vi "20260313_BIOEN468_FinalDraft_Final.vi"() -> ()   [LabVIEW 2025]
uses:
  <vilib>/Analysis/NI_AAL_SigProc.lvlib
  <vilib>/Waveform/WDTOps.llb/WDT Get Waveform Subset DBL.vi
  <vilib>/express/express analysis/Spectral/Block/exnSpectralBlock spectral measurements power poly.vi
  <vilib>/express/express analysis/Spectral/XNode/ExpressSpectralMeasurementsBlockNode.xnode
  <vilib>/Analysis/NI_AALBase.lvlib
  <vilib>/Analysis/baseanly.llb/Mean (DBL).vi
  <vilib>/express/express analysis/Spectral/Block/exnSpectralBlock spectral measurements power WFM.vi
  <vilib>/Waveform/WDTOps.llb/WDT Get XY Value DBL.vi
panel:
  out "Array 2":dbl[](array[numeric])
  out "Array":dbl[](array[numeric])
  out "Post truncation filtered top power spectrum":dbl[](graph)
  out "Post truncation filtered bottom power spectrum":dbl[](graph)
  out "Adventitious Lung Sound Detected":bool
  in  "threshold":dbl format="%.8f"
  out "# found":i32
  out "Bottom magnitudes":dbl[](graph)
  out "Top magnitudes":dbl[](graph)
  out "Subtracted magnitudes":dbl[](graph)
  out "Final Subtracted Power Spectrum":dbl[](graph)
  out "Truncated Waveform Top":waveform(dbl)(graph)
  in  "duration(s)  bottom":dbl
  out "sample rate (S/s) 2":dbl
  in  "File bottom":path
  in  "File top":path
  out "sample rate (S/s) 3":dbl
  in  "stop":bool
  in  "duration(s) top":dbl
  out "Truncated Waveform Bottom":waveform(dbl)(graph)
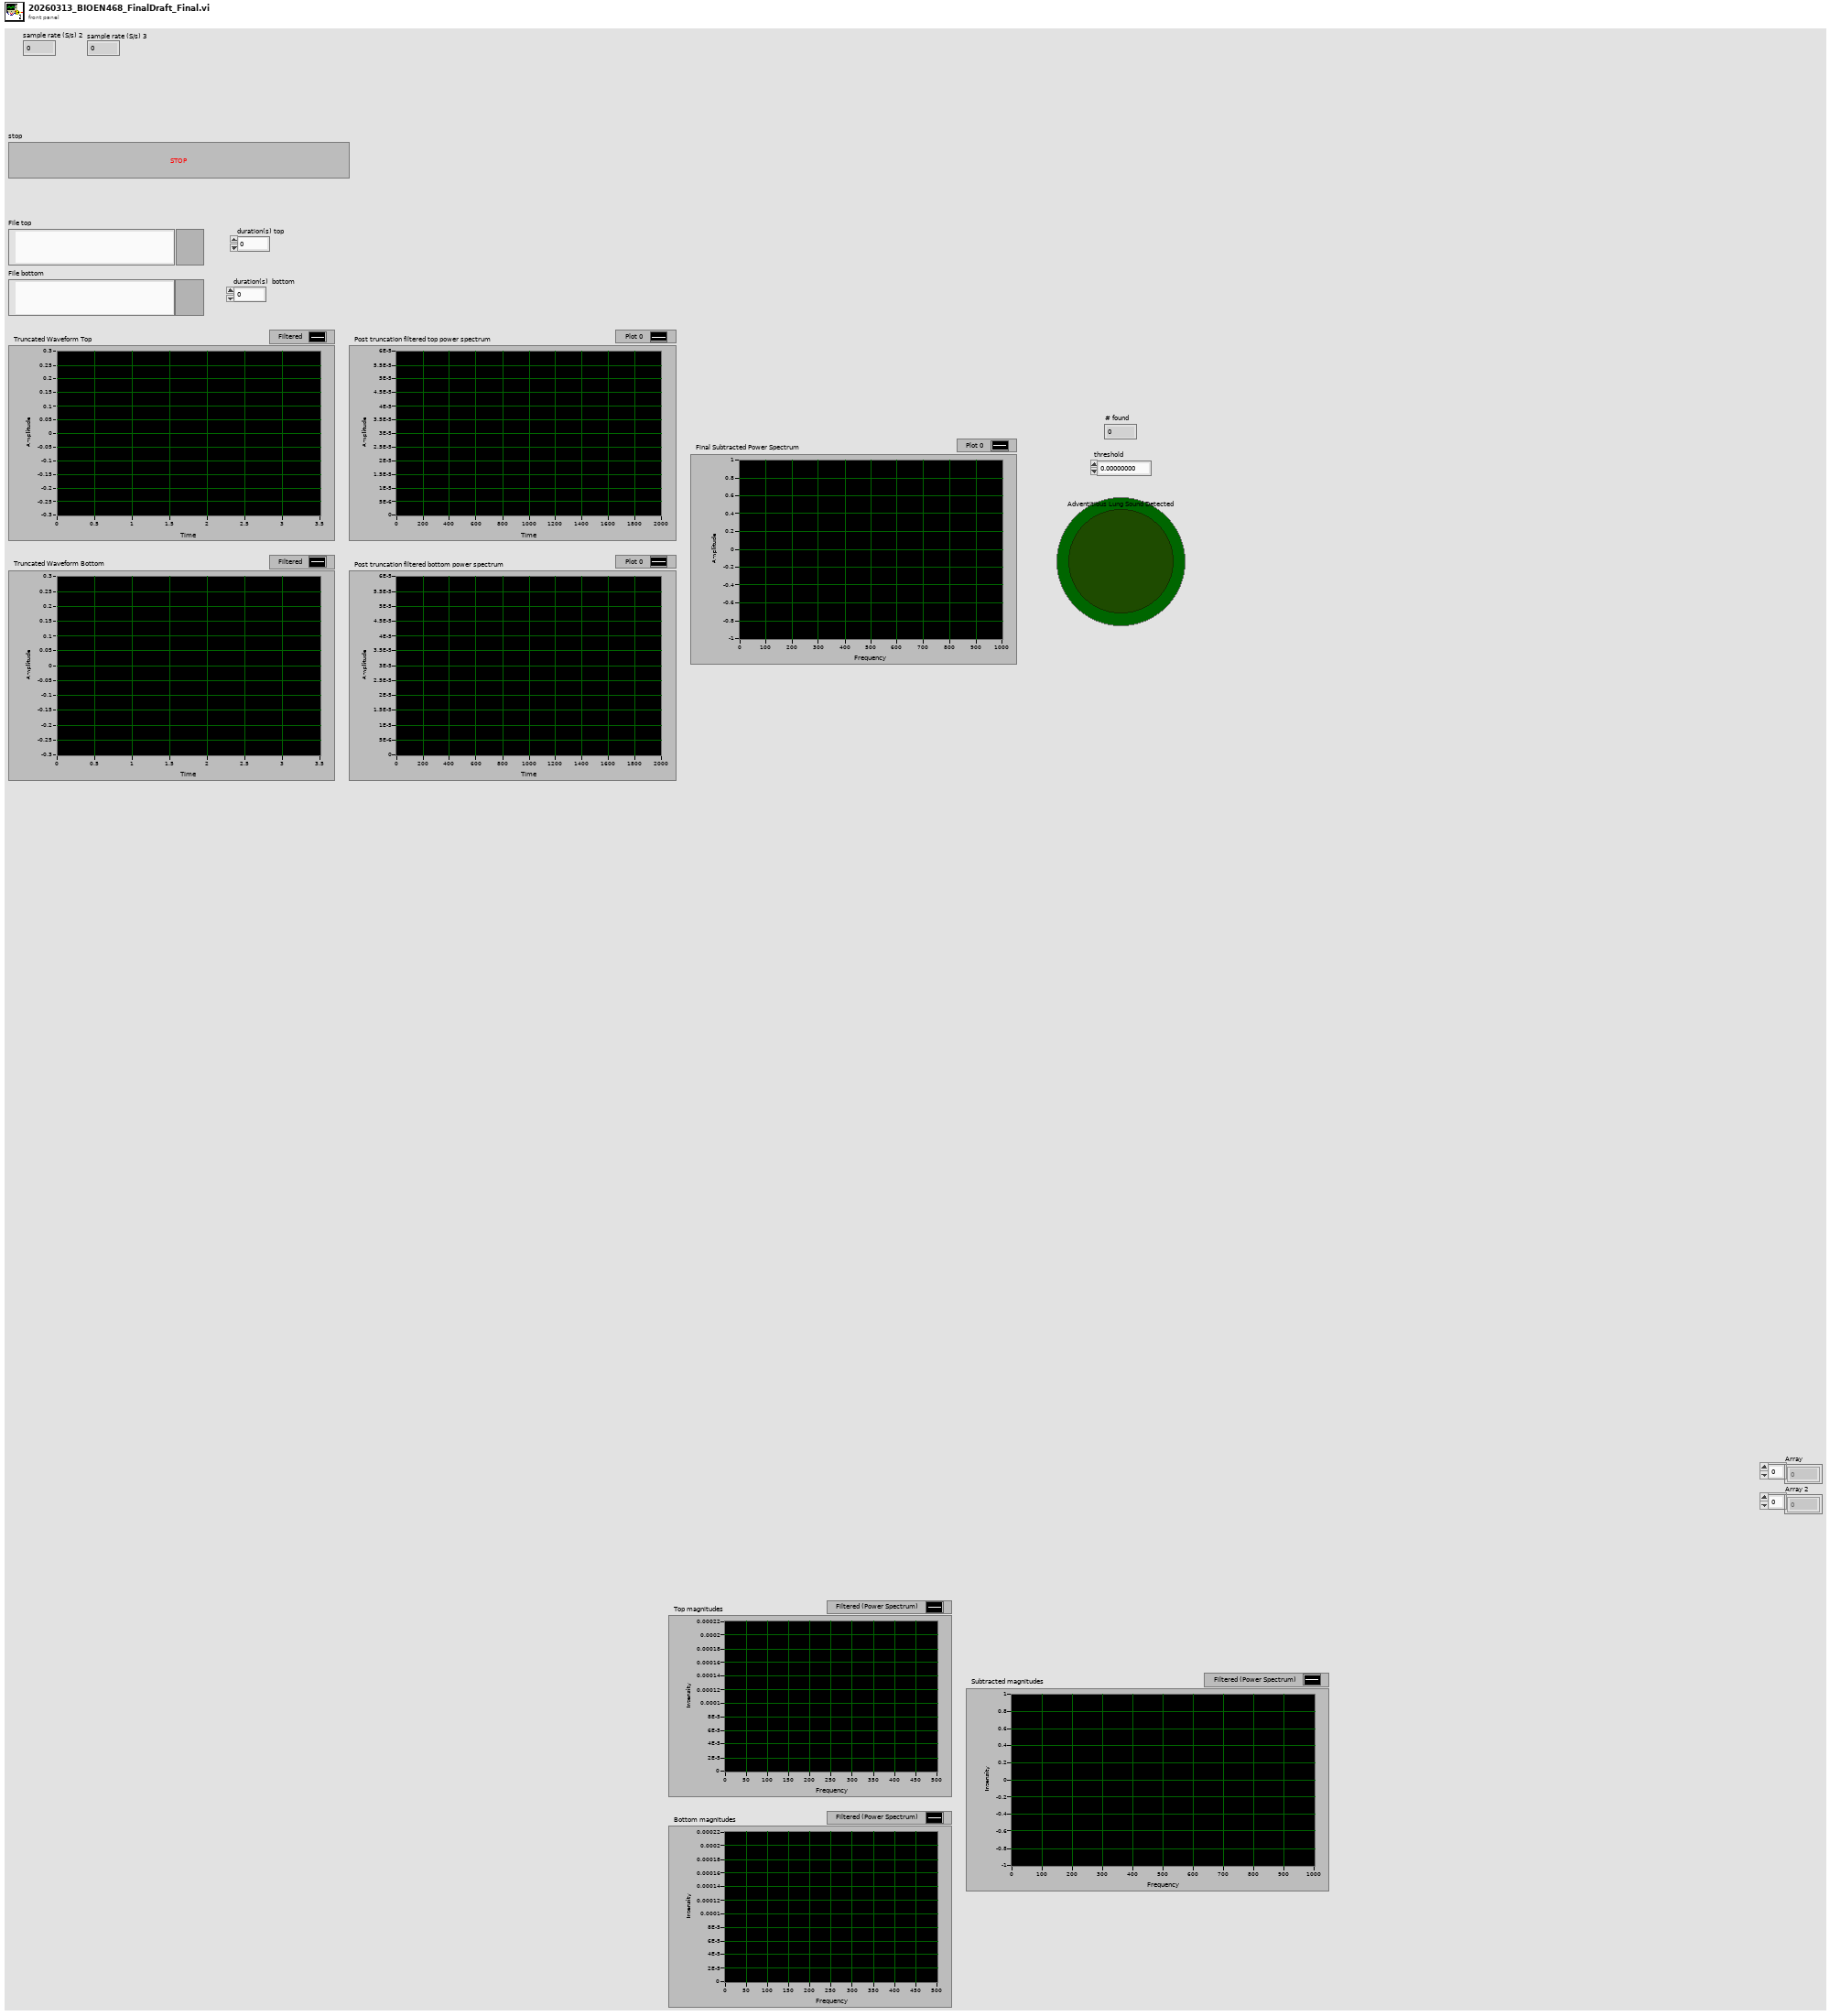
[diagram p1: front panel]
types:
  T1 = cluster{"averaging mode":u16, "weighting mode":u16, "number of averages":u32}
  T2 = cluster{"dB On (F)":bool, "unwrap phase (F)":bool, "convert to degree (F)":bool}
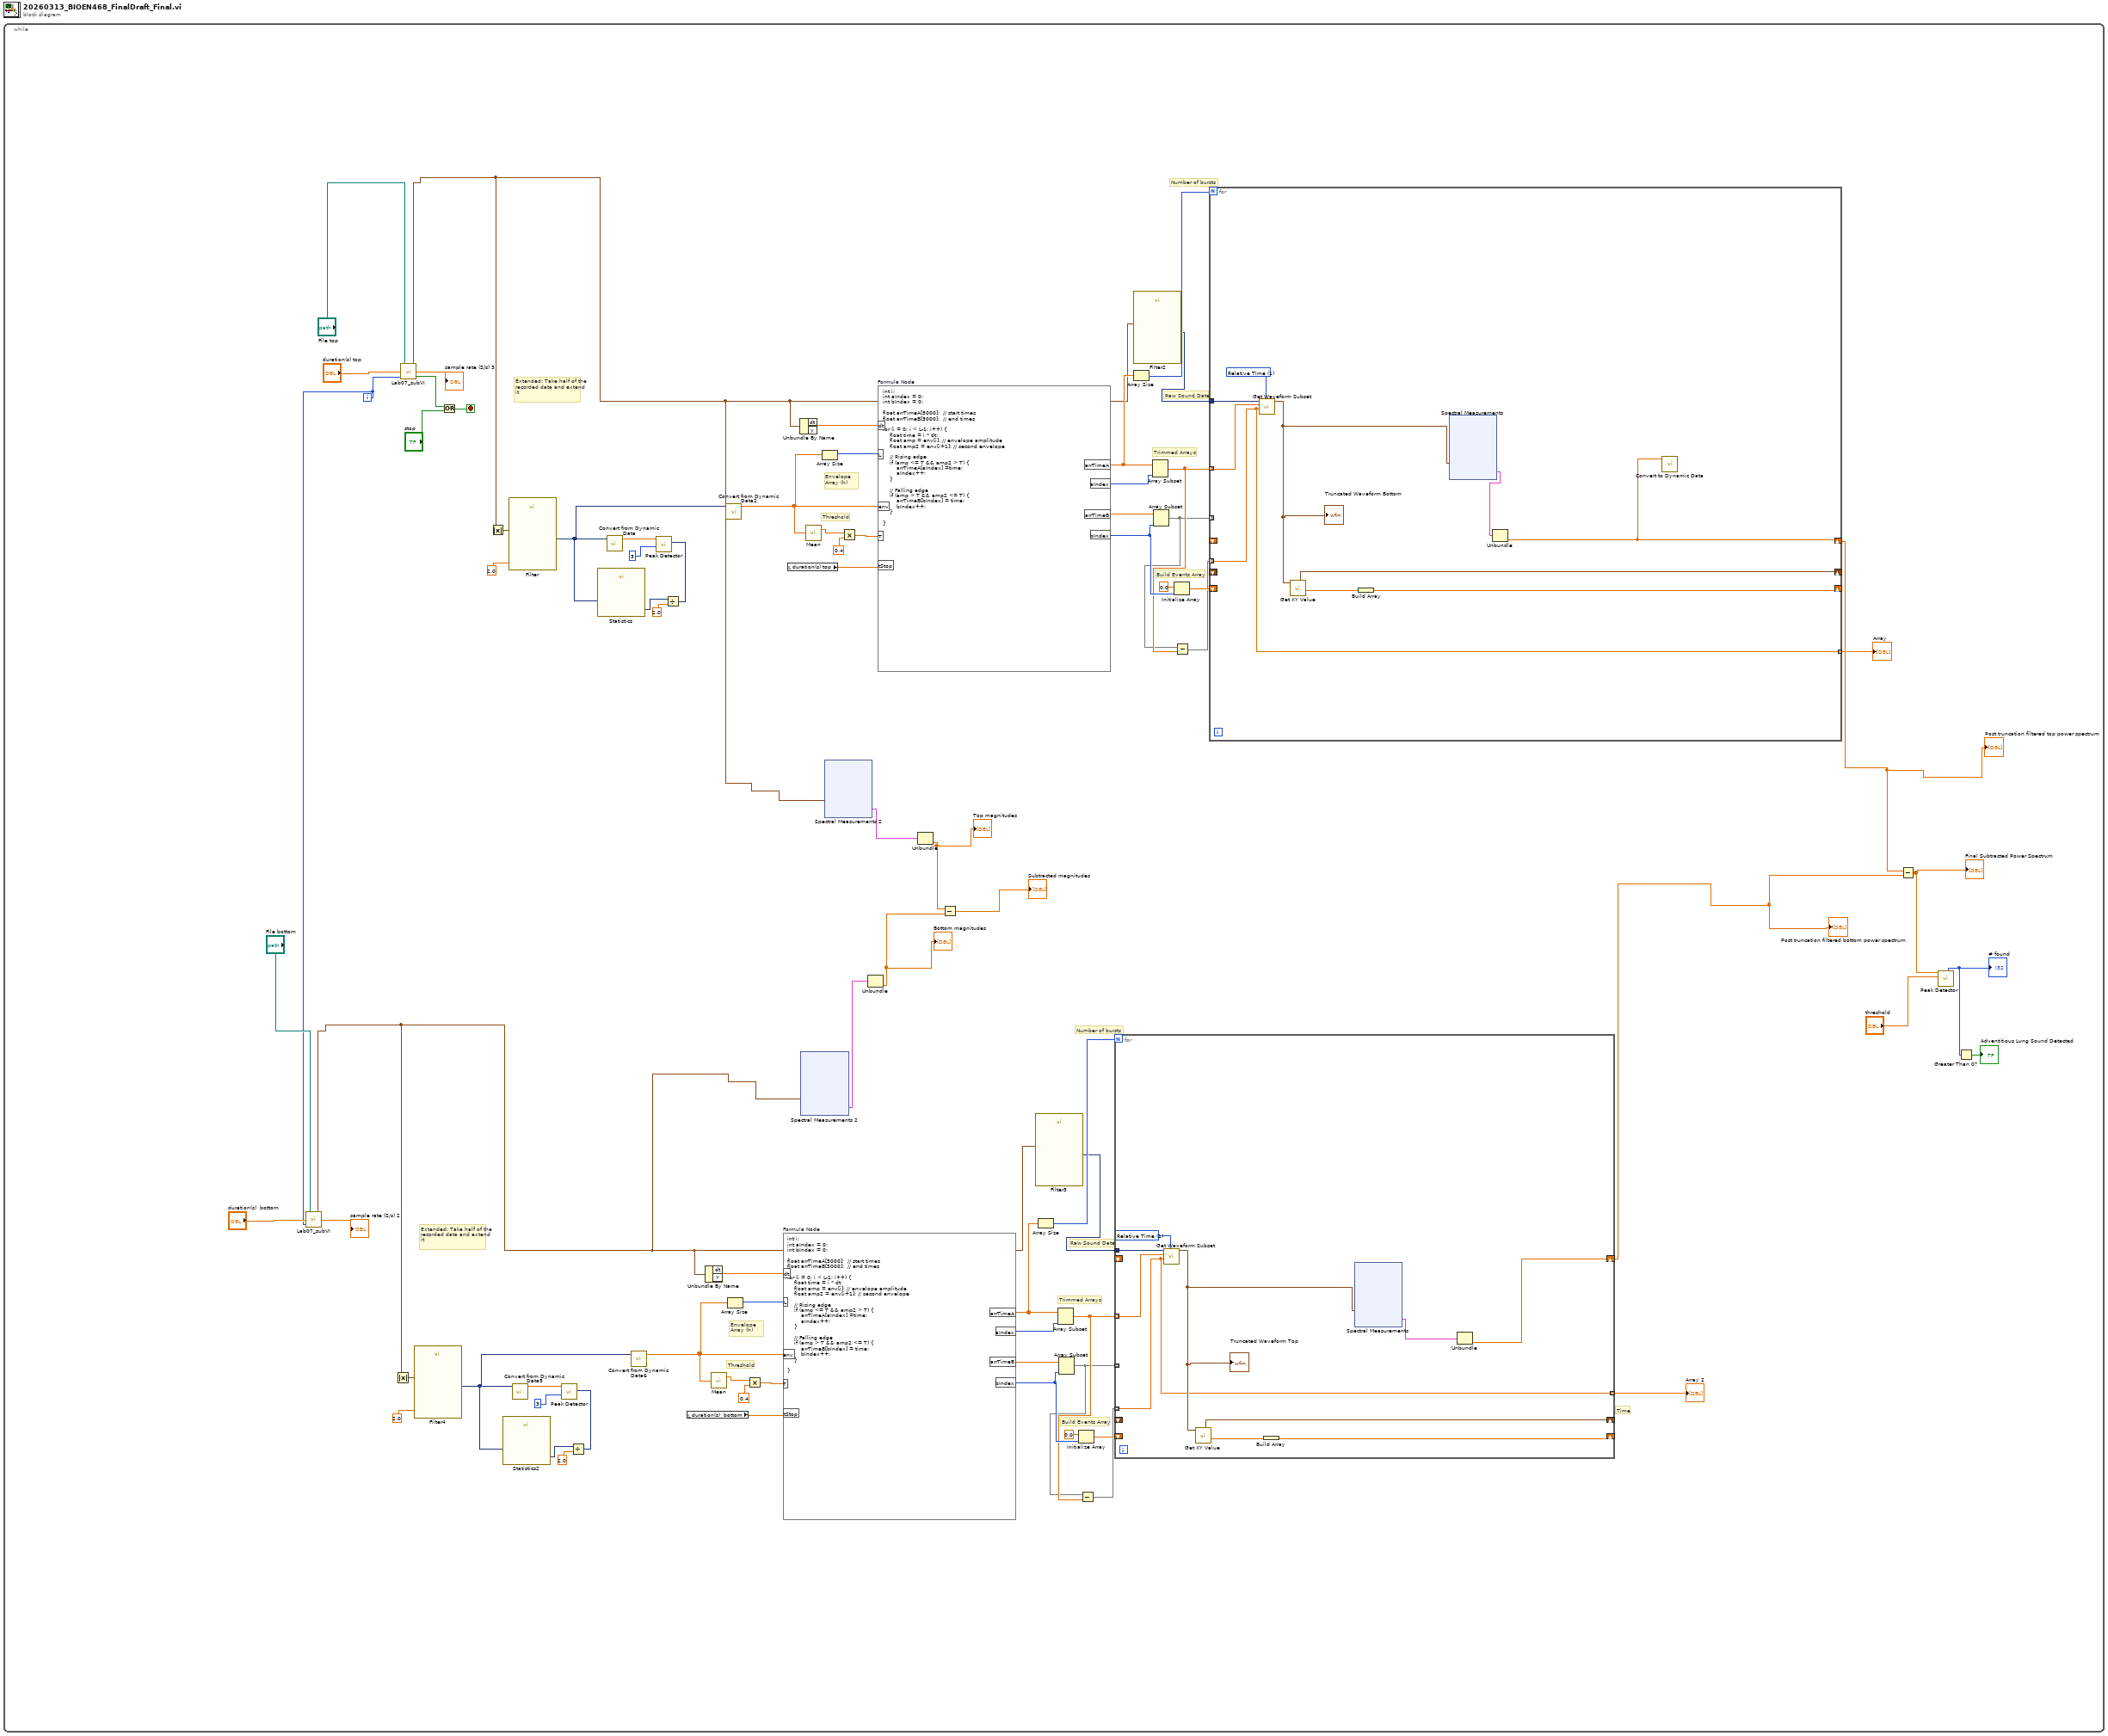
[diagram p0: block diagram]
diagram:
  n1 = while {
    i -> [w18]
    stop <- w73 stop-if-true
    # "Time"
    # "Build Events Array"
    # "Trimmed Arrays"
    # "Number of bursts"
    # "Raw Sound Data"
    # "Threshold"
    # "Envelope Array (h)"
    # "Extended: Take half of the recorded data and extend it"
    # "Build Events Array"
    # "Trimmed Arrays"
    # "Number of bursts"
    # "Raw Sound Data"
    # "Threshold"
    # "Envelope Array (h)"
    # "Extended: Take half of the recorded data and extend it"
    n2 = call "Lab07_subVI.vi"("i"=w18, "duration(s)"="duration(s)  bottom", "path"="File bottom") -> ("sample rate (S/s)"=→"sample rate (S/s) 2":dbl, "Waveform Segment"=w6:waveform(dbl))  [unwired: 1 out]
    n3 = Absolute Value(x=w6) -> (abs(x)=w43:waveform(dbl))
    n4 = call "Lab07_subVI.vi"("i"=w18, "duration(s)"="duration(s) top", "path"="File top") -> ("end of signal"=w75:bool, "sample rate (S/s)"=→"sample rate (S/s) 3":dbl, "Waveform Segment"=w8:waveform(dbl))
    n5 = call "Filter4"("Lower Cut-Off"=2.0, "Signal"=w43) -> ("Filtered Signal"=w37:dynamicdata)  [unwired: 8 in, 1 out]
    n6 = Or(x=w75, y="stop") -> (x .or. y?=w73:bool)
    n7 = Absolute Value(x=w8) -> (abs(x)=w71:waveform(dbl))
    n8 = call "Statistics2"("Signals"=w37) -> ("Maximum"=w40:dynamicdata)  [unwired: 25 in, 1 out]
    n9 = call "Filter"("Lower Cut-Off"=2.0, "Signal"=w71) -> ("Filtered Signal"=w65:dynamicdata)  [unwired: 8 in, 1 out]
    n10 = call "Convert from Dynamic Data5"("Dynamic Data Type"=w37) -> ("Array"=w42:dbl[])  [unwired: 3 in]
    n11 = Divide(x=w40, y=2.0) -> (x/y=w38:dynamicdata)
    n12 = call <vilib>:"Peak Detector.vi"("width"=3, "threshold"=w38, "X"=w42) -> ()  [unwired: 4 in, 5 out]
    n13 = call "Statistics"("Signals"=w65) -> ("Maximum"=w68:dynamicdata)  [unwired: 25 in, 1 out]
    n14 = call "Convert from Dynamic Data"("Dynamic Data Type"=w65) -> ("Array"=w70:dbl[])  [unwired: 3 in]
    n15 = call "Convert from Dynamic Data6"("Dynamic Data Type"=w37) -> ("Array"=w20:dbl[])  [unwired: 3 in]
    n16 = Divide(x=w68, y=2.0) -> (x/y=w66:dynamicdata)
    n17 = call <vilib>:"Peak Detector.vi"("width"=3, "threshold"=w66, "X"=w70) -> ()  [unwired: 4 in, 5 out]
    n18 = local read "duration(s)  bottom"() -> (w31:dbl)
    n19 = Unbundle By Name(w6) -> ("dt"=w30:dbl)  [unwired: 1 out]
    n20 = call-poly <vilib>:"Mean.vi"("X"=w20) -> ("mean"=w19:dbl)  [unwired: 1 out]
    n21 = call "Convert from Dynamic Data2"("Dynamic Data Type"=w65) -> ("Array"=w48:dbl[])  [unwired: 3 in]
    n22 = Array Size(array=w20) -> (size(s)=w34:i32)
    n23 = Multiply(x=w19, y=0.4) -> (x*y=w35:dbl)
    n24 = formula code="int i;\nint aIndex = 0;\nint bIndex = 0;\n\nfloat arrTimeA[5000];  // start times\nfloat arrTimeB[5000];  // end times\n\nfor (i = 0; i < L-1; i++) {\n    float time = i * dt;\n    float amp = env[i]; // envelope amplitude\n    float amp2 = env[i+1]; // second envelope\n\n    // Rising edge\n    if (amp <= T && amp2 > T) {\n        arrTimeA[aIndex] =time;\n        aIndex++;\n    }\n\n    // Falling edge\n    if (amp > T && amp2 <= T) {\n        arrTimeB[bIndex] = time;\n        bIndex++;\n    }\n\n}"("env"=w20, "T"=w35, "L"=w34, "tStop"=w31, "dt"=w30) -> ("arrTimeA"=w23:dbl[], "arrTimeB"=w25:dbl[], "aIndex"=w29:i32, "bIndex"=w28:i32)
    n25 = local read "duration(s) top"() -> (w59:dbl)
    n26 = Unbundle By Name(w8) -> ("dt"=w58:dbl)  [unwired: 1 out]
    n27 = xnode "Spectral Measurements 2"("Signals"=w6) -> ("Power Spectrum"=w16:cluster{"f0":dbl, "df":dbl, "magnitude":dbl[]})  [unwired: 1 in, 1 out]
    n28 = call-poly <vilib>:"Mean.vi"("X"=w48) -> ("mean"=w47:dbl)  [unwired: 1 out]
    n29 = Array Size(array=w48) -> (size(s)=w62:i32)
    n30 = xnode "Spectral Measurements 2"("Signals"=w8) -> ("Power Spectrum"=w17:cluster{"f0":dbl, "df":dbl, "magnitude":dbl[]})  [unwired: 1 in, 1 out]
    n31 = Multiply(x=w47, y=0.4) -> (x*y=w63:dbl)
    n32 = Unbundle(w16) -> ("magnitude"=w9:dbl[])  [unwired: 2 out]
    "Bottom magnitudes" <- w9
    n33 = formula code="int i;\nint aIndex = 0;\nint bIndex = 0;\n\nfloat arrTimeA[5000];  // start times\nfloat arrTimeB[5000];  // end times\n\nfor (i = 0; i < L-1; i++) {\n    float time = i * dt;\n    float amp = env[i]; // envelope amplitude\n    float amp2 = env[i+1]; // second envelope\n\n    // Rising edge\n    if (amp <= T && amp2 > T) {\n        arrTimeA[aIndex] =time;\n        aIndex++;\n    }\n\n    // Falling edge\n    if (amp > T && amp2 <= T) {\n        arrTimeB[bIndex] = time;\n        bIndex++;\n    }\n\n}"("env"=w48, "T"=w63, "L"=w62, "tStop"=w59, "dt"=w58) -> ("arrTimeA"=w51:dbl[], "arrTimeB"=w53:dbl[], "aIndex"=w57:i32, "bIndex"=w56:i32)
    n34 = Unbundle(w17) -> ("magnitude"=w14:dbl[])  [unwired: 2 out]
    "Top magnitudes" <- w14
    n35 = Subtract(x=w14, y=w9) -> (x-y=→"Subtracted magnitudes":dbl[])
    n36 = call "Filter3"("Signal"=w6) -> ("Filtered Signal"=w5:dynamicdata)  [unwired: 9 in, 1 out]
    n37 = Array Size(array=w23) -> (size(s)=w32:i32)
    n38 = Array Subset(array=w23, length=w29) -> (w22:dbl[])  [unwired: 1 in]
    n39 = Array Subset(array=w25, length=w28) -> (w21:dbl[])  [unwired: 1 in]
    n40 = Initialize Array(0.0 ("element"), w28) -> (w26:dbl[])
    n41 = Subtract(x=w21, y=w22) -> (x-y=w24:dbl[])
    n42 = for {
      N: w32 -> [_]
      tunnel: w5 -> [w96]
      tunnel: w24 -> [w87] mode=indexing
      tunnel: w22 -> [w95] mode=indexing
      tunnel: w21 -> [_] mode=indexing
      shift-right: [w92] -> _
      shift-left: w26 -> [_]
      shift-right: [w94] -> _
      shift-left: _ -> [_]
      shift-right: [w89] -> w3
      shift-left: _ -> [_]
      tunnel: [w87] -> w1 mode=indexing
      w91 = u16 1 items=["Samples", "Relative Time"] ("start/duration format")
      n43 = call-poly <vilib>:"Get Waveform Subset.vi"("start/duration format"=w91, "duration"=w87, "start samples/time"=w95, "waveform in"=w96) -> ("waveform out"=w88:waveform(dbl))  [unwired: 2 in, 3 out]
      "Truncated Waveform Top" <- w88
      n44 = call-poly <vilib>:"Get XY Value.vi"("waveform in"=w88) -> ("Y value"=w93:dbl, "X value"=w94:timestamp)  [unwired: 6 in, 3 out]
      n45 = Build Array(w93) -> (w92:dbl[])
      n46 = xnode "Spectral Measurements"("Signals"=w88) -> ("Power Spectrum"=w90:cluster{"f0":dbl, "df":dbl, "magnitude":dbl[]})  [unwired: 1 in, 1 out]
      n47 = Unbundle(w90) -> ("magnitude"=w89:dbl[])  [unwired: 2 out]
    }
    "Post truncation filtered bottom power spectrum" <- w3
    "Array 2" <- w1
    n48 = Array Size(array=w51) -> (size(s)=w60:i32)
    n49 = call "Filter2"("Signal"=w8) -> ("Filtered Signal"=w7:dynamicdata)  [unwired: 9 in, 1 out]
    n50 = Array Subset(array=w51, length=w57) -> (w50:dbl[])  [unwired: 1 in]
    n51 = Array Subset(array=w53, length=w56) -> (w49:dbl[])  [unwired: 1 in]
    n52 = Initialize Array(0.0 ("element"), w56) -> (w54:dbl[])
    n53 = Subtract(x=w49, y=w50) -> (x-y=w52:dbl[])
    n54 = for {
      N: w60 -> [_]
      tunnel: w7 -> [w124]
      tunnel: w52 -> [w115] mode=indexing
      tunnel: w50 -> [w123] mode=indexing
      tunnel: w49 -> [_] mode=indexing
      shift-right: [w120] -> _
      shift-left: w54 -> [_]
      shift-right: [w122] -> _
      shift-left: _ -> [_]
      shift-right: [w117] -> w4
      shift-left: _ -> [_]
      tunnel: [w115] -> w2 mode=indexing
      w119 = u16 1 items=["Samples", "Relative Time"] ("start/duration format")
      n55 = call-poly <vilib>:"Get Waveform Subset.vi"("start/duration format"=w119, "duration"=w115, "start samples/time"=w123, "waveform in"=w124) -> ("waveform out"=w116:waveform(dbl))  [unwired: 2 in, 3 out]
      "Truncated Waveform Bottom" <- w116
      n56 = call-poly <vilib>:"Get XY Value.vi"("waveform in"=w116) -> ("Y value"=w121:dbl, "X value"=w122:timestamp)  [unwired: 6 in, 3 out]
      n57 = Build Array(w121) -> (w120:dbl[])
      n58 = xnode "Spectral Measurements"("Signals"=w116) -> ("Power Spectrum"=w118:cluster{"f0":dbl, "df":dbl, "magnitude":dbl[]})  [unwired: 1 in, 1 out]
      n59 = Unbundle(w118) -> ("magnitude"=w117:dbl[])  [unwired: 2 out]
      n60 = call "Convert to Dynamic Data"("Array"=w117) -> ()  [unwired: 3 in, 1 out]
    }
    "Post truncation filtered top power spectrum" <- w4
    "Array" <- w2
    n61 = Subtract(x=w4, y=w3) -> (x-y=w13:dbl[])
    "Final Subtracted Power Spectrum" <- w13
    n62 = call <vilib>:"Peak Detector.vi"("threshold"="threshold", "X"=w13) -> ("# found"=w11:i32)  [unwired: 5 in, 4 out]
    "# found" <- w11
    n63 = Greater Than 0?(x=w11) -> (x > 0?=→"Adventitious Lung Sound Detected":bool)
  }
